vi "Format Fraction.vi"(3 "Den":i32, 5 "Num":i32) -> (0 "Pct":dbl, 2 "String (N/D)":string)   [LabVIEW 2015]
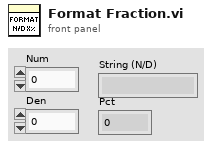
[diagram p1: front panel]
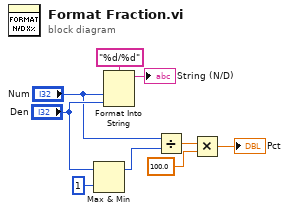
[diagram p0: block diagram]
diagram:
  n1 = Max & Min(x="Den", y=1) -> (max(x,y)=w7:i32)  [unwired: 1 out]
  n2 = Format Into String(format string="%d/%d" ("initial string"), "Num", "Den") -> (resulting string=→"String (N/D)":string)  [unwired: 2 in, 1 out]
  n3 = Divide(x="Num", y=w7) -> (x/y=w6:dbl)
  n4 = Multiply(x=w6, y=100.0) -> (x*y=→"Pct":dbl)
